vi "getConvertControl.vi"(8 "error in (no error)":errorcluster, 10 "data_format":T1(ring)=enum."Mono16", 11 "Camera in":refnum<class "Camera.lvclass">) -> (0 "error out":errorcluster, 2 "convert_control":T2={"sharpen"=TRUE, "adaptive_sharpen"=TRUE, "flip_vertical"=FALSE, "auto_minmax"=TRUE, "min_limit"=0, "max_limit"=20000, "gamma"=1.0, "contrast"=0, "pco_debayer_algorithm"=FALSE, "color_temperature"=6500, "color_saturation"=0, "color_vibrance"=0, "color_tint"=0, "lut_file"=path ""} {"gamma" format="%#_6f"}, 3 "Camera out":refnum<class "Camera.lvclass">)   [LabVIEW 2020, in "Camera.lvclass"]
doc: "Gets the current configuration from the camera."
uses:
  Camera.lvclass
  Camera.lvclass/Camera.ctl
  Convert.lvlib
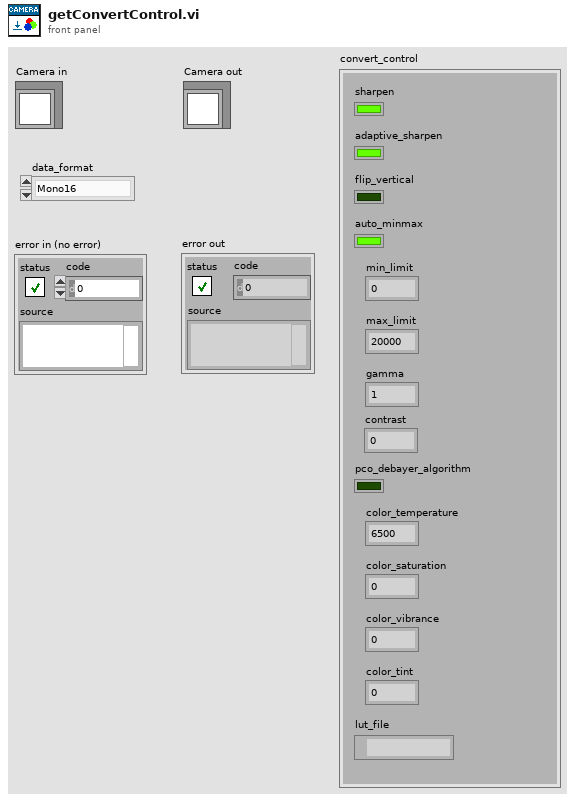
[diagram p1: front panel]
types:
  T1 = enum16{"Undefined", "Mono8", "Mono16", "BGRA8", "RGBA8", "BGRA16", "RGBA16", "CompressedMono8"}
  T2 = cluster{"sharpen":bool, "adaptive_sharpen":bool, "flip_vertical":bool, "auto_minmax":bool, "min_limit":u16, "max_limit":u16, "gamma":dbl, "contrast":i32, "pco_debayer_algorithm":bool, "color_temperature":i32, "color_saturation":i32, "color_vibrance":i32, "color_tint":i32, "lut_file":path}
  T3 = map{enum16{"Undefined", "Mono8", "Mono16", "BGRA8", "RGBA8", "BGRA16", "RGBA16", "CompressedMono8"}, cluster{"sharpen":bool, "adaptive_sharpen":bool, "flip_vertical":bool, "auto_minmax":bool, "min_limit":u16, "max_limit":u16, "gamma":dbl, "contrast":i32, "pco_debayer_algorithm":bool, "color_temperature":i32, "color_saturation":i32, "color_vibrance":i32, "color_tint":i32, "lut_file":path}}
  T4 = cluster{"wScale_minmax":u16, "iScale_maxmax":i32, "iScale_min":i32, "iScale_max":i32, "iColor_temp":i32, "iColor_tint":i32, "iColor_saturation":i32, "iColor_vibrance":i32, "iContrast":i32, "iGamma":i32, "iSRGB":i32, "pHistogramData":u64, "dwProcessingFlags":u32, "wProzValue4Min":u16, "wProzValue4Max":u16}
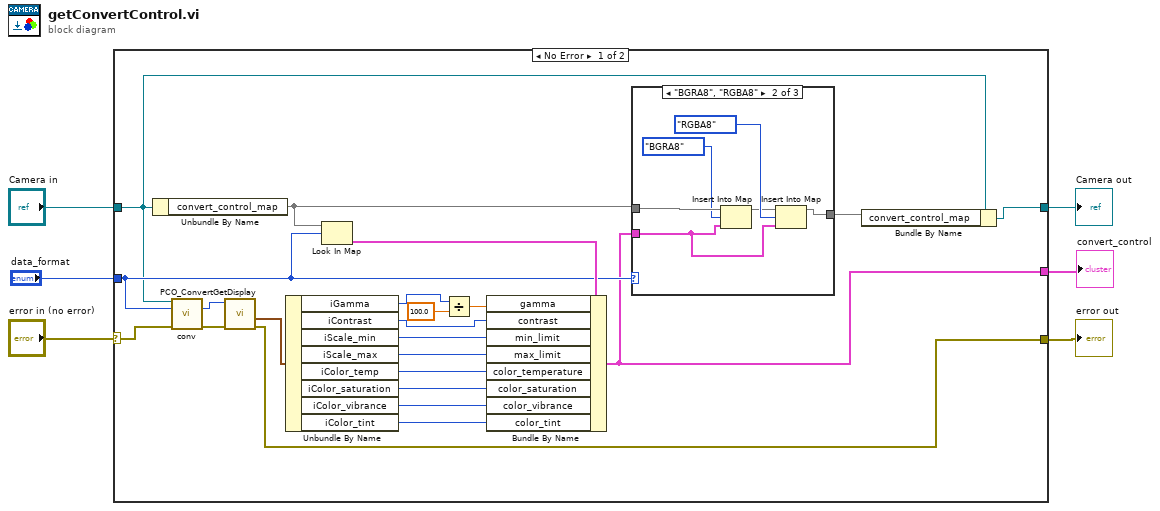
[diagram p0: block diagram]
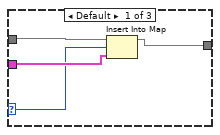
[diagram p2: hidden frame]
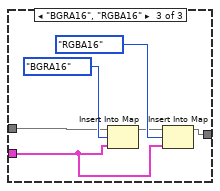
[diagram p3: hidden frame]
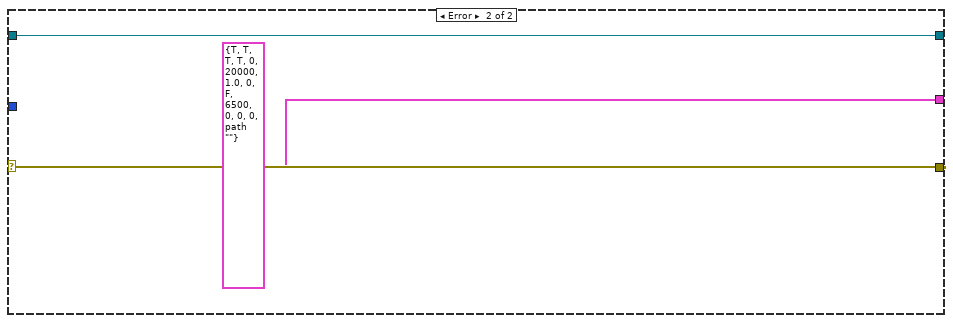
[diagram p4: hidden frame]
diagram:
  n1 = case shown="No Error" "error in (no error)" {
    selector: "error in (no error)" -> [w28 w47]
    tunnel: [w10 w47] -> w5
    tunnel: [w7 w46] -> w3
    tunnel: "Camera in" -> [w9 w46]
    tunnel: [w11 T2 {"sharpen"=TRUE, "adaptive_sharpen"=TRUE, "flip_vertical"=TRUE, "auto_minmax"=TRUE, "min_limit"=0, "max_limit"=20000, "gamma"=1.0, "contrast"=0, "pco_debayer_algorithm"=FALSE, "color_temperature"=6500, "color_saturation"=0, "color_vibrance"=0, "color_tint"=0, "lut_file"=path ""} ("convert_control")] -> w2
    tunnel: "data_format" -> [w13 _]
    frame No Error {
      n2 = Unbundle By Name(w9) -> ("convert_control_map"=w12:T3)
      n3 = call-dynamic "conv.vi"("Camera in"=w9, "data_format"=w13, "error in (no error)"=w28) -> ("conv"=w26:u64, "error out"=w27:errorcluster)  [unwired: 10 in, 1 out]
      n4 = call "PCO_ConvertGetDisplay.vi"("error in (no error)"=w27, "ph"=w26) -> ("error out"=w10:errorcluster, "strDisplay"=w24:T4)  [unwired: 6 in, 2 out]
      n5 = Unbundle By Name(w24) -> ("iGamma"=w21:i32, "iContrast"=w20:i32, "iScale_min"=w19:i32, "iScale_max"=w18:i32, "iColor_temp"=w17:i32, "iColor_saturation"=w16:i32, "iColor_vibrance"=w15:i32, "iColor_tint"=w14:i32)
      n6 = Look In Map(map=w12, key=w13) -> (value=w25:T2)  [unwired: 1 in, 1 out]
      n7 = Divide(x=w21, y=100.0) -> (x/y=w23:dbl)
      n8 = Bundle By Name(cluster=w25, "gamma"=w23, "contrast"=w20, "min_limit"=w19, "max_limit"=w18, "color_temperature"=w17, "color_saturation"=w16, "color_vibrance"=w15, "color_tint"=w14) -> (w11:T2)
      n9 = case shown="\"BGRA8\", \"RGBA8\"" w13 {
        selector: w13 -> [w30 _ _]
        tunnel: w12 -> [w31 w38 w40]
        tunnel: w11 -> [w32 w36 w39]
        tunnel: [w29 w33 w41] -> w8
        frame Default {
          n10 = Insert Into Map(map in=w31, key=w30, value=w32) -> (map out=w29:T3)  [unwired: 2 out]
        }
        frame "BGRA8", "RGBA8" {
          n11 = Insert Into Map(map in=w38, key=T1."BGRA8" ("data_format"), value=w36) -> (map out=w34:T3)  [unwired: 2 out]
          n12 = Insert Into Map(map in=w34, key=T1."RGBA8" ("data_format"), value=w36) -> (map out=w33:T3)  [unwired: 2 out]
        }
        frame "BGRA16", "RGBA16" {
          n13 = Insert Into Map(map in=w40, key=T1."BGRA16" ("data_format"), value=w39) -> (map out=w42:T3)  [unwired: 2 out]
          n14 = Insert Into Map(map in=w42, key=T1."RGBA16" ("data_format"), value=w39) -> (map out=w41:T3)  [unwired: 2 out]
        }
      }
      n15 = Bundle By Name(cluster=w9, "convert_control_map"=w8) -> (w7:refnum<class "Camera.lvclass">)
    }
    frame Error {
    }
  }
  "error out" <- w5
  "Camera out" <- w3
  "convert_control" <- w2
